vi "Teleop.vi"(10 "Match Info":T1={"Autonomous Elapsed Seconds"=0.0, "TeleOp Elapsed Seconds"=0.0, "Disabled Elapsed Seconds"=0.0, "Visited Autonomous"=FALSE, "Visited TeleOp"=FALSE, "Visited Disabled"=FALSE, "Autonomous Settings"={"Autonomous Style"=enum."Independent", "VI Refnum"=refnum}}, 11 "Call Context":T2) -> ()   [LabVIEW 2014]
doc: "This VI is called for each TeleOp packet received from the DS where the robot is not disabled. It is often used to read from the joysticks and update I/O or to update setpoints for timed control loops. It should complete and return within 20 milliseconds or it may miss DS packets."
uses:
  <vilib>/Rock Robotics/Network Tables/SD Write Numeric Array.vi
  <vilib>/Rock Robotics/Network Tables/SD Read Boolean.vi
  <vilib>/Rock Robotics/Network Tables/SD Read Number.vi
  <vilib>/Rock Robotics/Network Tables/SD Write Boolean Array.vi
  <vilib>/Rock Robotics/WPI/DriverStation/WPI_DriverStationMatch Info.ctl
  <vilib>/Rock Robotics/WPI/DriverStation/WPI_DriverStationDerivedRobotMode.ctl
panel:
  out "Sample Slider 0":dbl(slide) scale=0.0..5.0
  out "Sample Boolean 1":bool
  out "Sample Boolean 0":bool
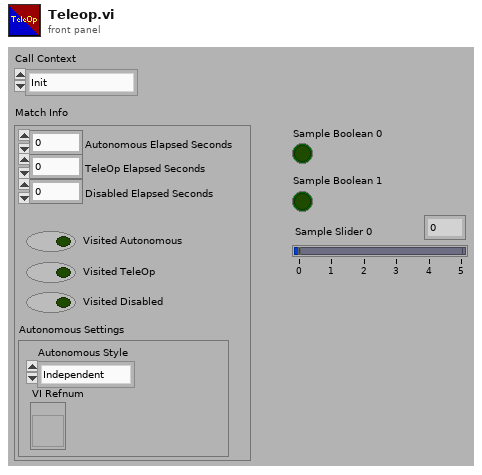
[diagram p1: front panel]
types:
  T1 = typedef "WPI_DriverStationMatch Info.ctl" = cluster{"Autonomous Elapsed Seconds":dbl, "TeleOp Elapsed Seconds":dbl, "Disabled Elapsed Seconds":dbl, "Visited Autonomous":bool, "Visited TeleOp":bool, "Visited Disabled":bool, "Autonomous Settings":cluster{"Autonomous Style":enum16{"Iterative", "Independent"}, "VI Refnum":refnum<vi>}}
  T2 = typedef "WPI_DriverStationDerivedRobotMode.ctl" = enum16{"Init", "Execute", "Stop"}
  T3 = typedef "WPI_RobotDriveDevRef.ctl" = cluster{"DevStatus":errorcluster, "Motors[]":T4[], "Square Inputs":bool, "Max Output":dbl}
  T4 = typedef "WPI_MotorControlDeviceRef.ctl" = cluster{"DeviceStatus":errorcluster, "Type":T5, "PWM":cluster{"Controller":T6, "PWM Channel":T7, "DeadBand":T8}, "CAN":cluster{"Device Number":u8, "Control Mode":T9, "Semaphore":T10, "Max Vout":dbl, "TalonSRX Control Mode":T11}, "Invert":bool, "TransformRef":T12, "InvTransformRef":T12}
  T5 = typedef "WPI_MotorControlType.ctl" = enum16{"PWM", "CAN", "CANTalonSRX"}
  T6 = typedef "FPGA_TypedefDigitalModule.ctl" = enum16{"Controller 1"}
  T7 = typedef "FPGA_DIOPWMChannel.ctl" = enum8{"PWM 0", "PWM 1", "PWM 2", "PWM 3", "PWM 4", "PWM 5", "PWM 6", "PWM 7", "PWM 8", "PWM 9", "PWM MXP 0", "PWM MXP 1", "PWM MXP 2", "PWM MXP 3", "PWM MXP 4", "PWM MXP 5", "PWM MXP 6", "PWM MXP 7", "PWM MXP 8", "PWM MXP 9", "Invalid"}
  T8 = typedef "WPI_PWMDeadband.ctl" = cluster{"Name":string, "maxPositivePwm":i32, "minPositivePwm":i32, "centerPwm":i32, "maxNegativePwm":i32, "minNegativePwm":i32, "angularRange":u16}
  T9 = typedef "WPI_CANJaguar_ControlMode.ctl" = enum8{"Percent VBus", "Current", "Speed", "Position", "Voltage"}
  T10 = typedef "Semaphore RefNum" = refnum<k1>
  T11 = typedef "WPI_CANTalonSRX_APIControlMode.ctl" = enum8{"Percent VBus", "Speed", "Position", "Slave", "Unchanged / Invalid"}
  T12 = typedef "WPI_PWMTransform_ConPane.ctl" = refnum<vi>
  T13 = typedef "WPI_JoystickDevRef.ctl" = cluster{"Device":T14}
  T14 = typedef "WPI_JoystickDeviceEnum.ctl" = enum16{"USB 0", "USB 1", "USB 2", "USB 3", "USB 4", "USB 5"}
  T15 = typedef "WPI_PotentiometerDevRef.ctl" = cluster{"DevStatus":errorcluster, "Controller":T16, "Analog Channel":T17, "Invert Output":bool}
  T16 = typedef "FPGA_TypedefAnalogModule.ctl" = enum16{"Controller 1"}
  T17 = typedef "FPGA_AIChannel.ctl" = enum8{"AI 0", "AI 1", "AI 2", "AI 3", "AI MXP 0", "AI MXP 1", "AI MXP 2", "AI MXP 3", "Invalid"}
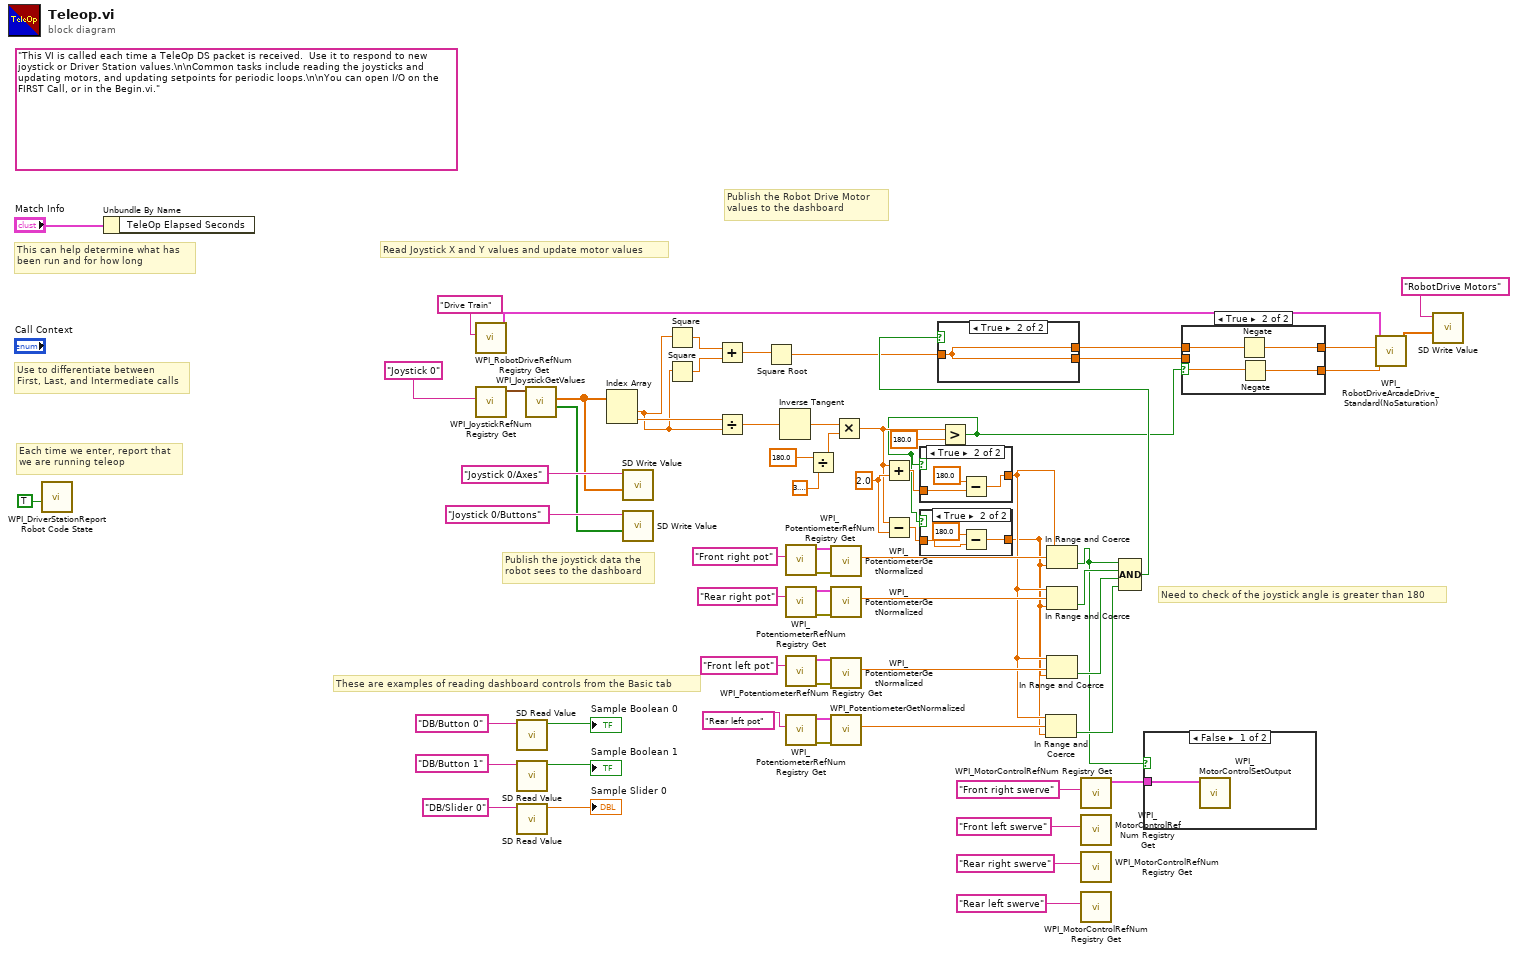
[diagram p0: block diagram]
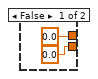
[diagram p6: hidden frame]
diagram:
  w47 = 2.0 ("y")
  (unwired) "This VI is called each time a TeleOp DS packet is received.  Use it to respond to new joystick or Driver Station values.\n\nCommon tasks include reading the joysticks and updating motors, and updating setpoints for periodic loops.\n\nYou can open I/O on the FIRST Call, or in the Begin.vi."
  # "Need to check of the joystick angle is greater than 180"
  # "These are examples of reading dashboard controls from the Basic tab"
  # "Publish the Robot Drive Motor\nvalues to the dashboard"
  # "Publish the joystick data the\nrobot sees to the dashboard"
  # "Each time we enter, report that\nwe are running teleop"
  # "Use to differentiate between\nFirst, Last, and Intermediate calls"
  # "This can help determine what has\nbeen run and for how long"
  # "Read Joystick X and Y values and update motor values"
  n1 = call <vilib>:"WPI_DriverStationReport Robot Code State.vi"("TeleOp"=TRUE ("Autonomous")) -> ()  [unwired: 10 in, 1 out]
  n2 = Unbundle By Name("Match Info") -> ()  [unwired: 1 out]
  n3 = call <vilib>:"WPI_RobotDriveRefNum Registry Get.vi"("refnum name"="Drive Train") -> ("RobotDriveDevRef"=w66:T3)  [unwired: 1 in, 9 out]
  n4 = call <vilib>:"WPI_JoystickRefNum Registry Get.vi"("refnum name"="Joystick 0") -> ("JoystickDevRef"=w64:T13)  [unwired: 1 in, 9 out]
  n5 = call-poly <vilib>:"SD Read Value.vi"("Name"="DB/Button 0" ("refnum name")) -> ("Boolean"=→"Sample Boolean 0":bool)  [unwired: 8 in, 2 out]
  n6 = call-poly <vilib>:"SD Read Value.vi"("Name"="DB/Button 1" ("refnum name")) -> ("Boolean"=→"Sample Boolean 1":bool)  [unwired: 8 in, 2 out]
  n7 = call-poly <vilib>:"SD Read Value.vi"("Name"="DB/Slider 0" ("refnum name")) -> ("Numeric"=→"Sample Slider 0":dbl)  [unwired: 8 in, 2 out]
  n8 = call <vilib>:"WPI_JoystickGetValues.vi"("JoystickDevRef"=w64) -> ("Buttons"=w51:bool[], "Axes"=w53:dbl[])  [unwired: 6 in, 3 out]
  n9 = Index Array(array=w53) -> (element #1=w30:dbl, element #2=w32:dbl)  [unwired: 2 in]
  n10 = call-poly <vilib>:"SD Write Value.vi"("Numeric Array"=w53, "Name"="Joystick 0/Axes") -> ()  [unwired: 8 in, 2 out]
  n11 = call-poly <vilib>:"SD Write Value.vi"("Boolean Array"=w51, "Name"="Joystick 0/Buttons") -> ()  [unwired: 8 in, 2 out]
  n12 = Square(x=w30) -> (x^2=w29:dbl)
  n13 = Square(x=w30) -> (x^2=w28:dbl)
  n14 = Add(x=w29, y=w28) -> (x+y=w27:dbl)
  n15 = Divide(x=w32, y=w30) -> (x/y=w48:dbl)
  n16 = Square Root(x=w27) -> (sqrt(x)=w26:dbl)
  n17 = Inverse Tangent(1:w48) -> (0:w19:dbl)
  n18 = call <vilib>:"WPI_PotentiometerRefNum Registry Get.vi"("refnum name"="Front right pot") -> ("error out"=w46:errorcluster, "PotDevRef"=w45:T15)  [unwired: 9 in]
  n19 = call <vilib>:"WPI_PotentiometerRefNum Registry Get.vi"("refnum name"="Rear right pot") -> ("error out"=w35:errorcluster, "PotDevRef"=w34:T15)  [unwired: 9 in]
  n20 = call <vilib>:"WPI_PotentiometerRefNum Registry Get.vi"("refnum name"="Front left pot") -> ("error out"=w42:errorcluster, "PotDevRef"=w41:T15)  [unwired: 9 in]
  n21 = call <vilib>:"WPI_PotentiometerRefNum Registry Get.vi"("refnum name"="Rear left pot") -> ("error out"=w38:errorcluster, "PotDevRef"=w37:T15)  [unwired: 9 in]
  n22 = Divide(x=180.0, y=3.141592653589793) -> (x/y=w16:dbl)
  n23 = call <vilib>:"WPI_PotentiometerGetNormalized.vi"("error in"=w46, "PotDevRef"=w45) -> ("Normalized Value"=w9:dbl)  [unwired: 7 in, 2 out]
  n24 = call <vilib>:"WPI_PotentiometerGetNormalized.vi"("error in"=w35, "PotDevRef"=w34) -> ("Normalized Value"=w8:dbl)  [unwired: 7 in, 2 out]
  n25 = call <vilib>:"WPI_PotentiometerGetNormalized.vi"("error in"=w42, "PotDevRef"=w41) -> ("Normalized Value"=w7:dbl)  [unwired: 7 in, 2 out]
  n26 = call <vilib>:"WPI_PotentiometerGetNormalized.vi"("error in"=w38, "PotDevRef"=w37) -> ("Normalized Value"=w6:dbl)  [unwired: 7 in, 2 out]
  n27 = Multiply(x=w19, y=w16) -> (x*y=w15:dbl)
  n28 = Add(x=w15, y=w47) -> (x+y=w5:dbl)
  n29 = Subtract(x=w15, y=w47) -> (x-y=w3:dbl)
  n30 = Greater?(x=w15, y=180.0) -> (0:w2:bool)
  n31 = case shown="True" w2 {
    tunnel: w5 -> [w68 w70]
    tunnel: [w68 w69] -> w4
    frame False {
    }
    frame True {
      n32 = Subtract(x=180.0, y=w70) -> (x-y=w69:dbl)
    }
  }
  n33 = case shown="True" w2 {
    tunnel: w3 -> [_ w73]
    tunnel: [_ w72] -> w1
    frame False {
    }
    frame True {
      n34 = Subtract(x=180.0, y=w73) -> (x-y=w72:dbl)
    }
  }
  n35 = In Range and Coerce(upper limit=w4, x=w6, lower limit=w1) -> (In Range?=w39:bool)  [unwired: 1 out]
  n36 = In Range and Coerce(upper limit=w4, x=w9, lower limit=w1) -> (In Range?=w21:bool)  [unwired: 1 out]
  n37 = In Range and Coerce(upper limit=w4, x=w8, lower limit=w1) -> (In Range?=w49:bool)  [unwired: 1 out]
  n38 = In Range and Coerce(upper limit=w4, x=w7, lower limit=w1) -> (In Range?=w43:bool)  [unwired: 1 out]
  n39 = call <vilib>:"WPI_MotorControlRefNum Registry Get.vi"("refnum name"="Front right swerve") -> ("MotorControlDevRef"=w20:T4)  [unwired: 9 in, 1 out]
  n40 = call <vilib>:"WPI_MotorControlRefNum Registry Get.vi"("refnum name"="Front left swerve") -> ()  [unwired: 9 in, 2 out]
  n41 = call <vilib>:"WPI_MotorControlRefNum Registry Get.vi"("refnum name"="Rear right swerve") -> ()  [unwired: 9 in, 2 out]
  n42 = call <vilib>:"WPI_MotorControlRefNum Registry Get.vi"("refnum name"="Rear left swerve") -> ()  [unwired: 9 in, 2 out]
  n43 = Compound Arithmetic op=AND(w21, w49, w43, w39) -> (w31:bool)
  n44 = case shown="True" w31 {
    tunnel: [0.0 w77] -> w13
    tunnel: [0.0 w77] -> w12
    tunnel: w26 -> [_ w77]
    frame False {
    }
    frame True {
    }
  }
  n45 = case shown="False" w21 {
    tunnel: w20 -> [w78 _]
    frame False {
      n46 = call <vilib>:"WPI_MotorControlSetOutput.vi"("MotorControlDevRef"=w78) -> ()  [unwired: 8 in, 3 out]
    }
    frame True {
    }
  }
  n47 = case shown="True" w2 {
    tunnel: w13 -> [w80 w84]
    tunnel: w12 -> [w79 w83]
    tunnel: [w79 w82] -> w10
    tunnel: [w80 w81] -> w11
    frame False {
    }
    frame True {
      n48 = Negate(x=w84) -> (-x=w81:dbl)
      n49 = Negate(x=w83) -> (-x=w82:dbl)
    }
  }
  n50 = call <vilib>:"WPI_RobotDriveArcadeDrive_Standard(NoSaturation).vi"("Y axis value"=w10, "X axis value"=w11, "RobotDriveDevRef"=w66) -> ("Motor Values"=w55:dbl[])  [unwired: 1 in, 7 out]
  n51 = call-poly <vilib>:"SD Write Value.vi"("Numeric Array"=w55, "Name"="RobotDrive Motors") -> ()  [unwired: 8 in, 2 out]
